vi "Factorial.vi"() -> ()   [LabVIEW 2022 SP3]
panel:
  out "N!":i64
  in  "N":i32
  # "Factorial:\nEnter a number N, to see the value of N!\nWhere N! = 1 * 2 * 3 * 4 * ... * N"
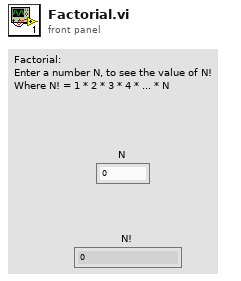
[diagram p1: front panel]
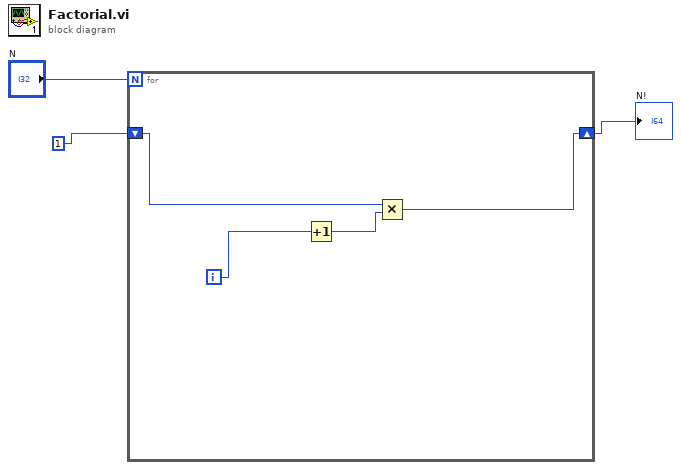
[diagram p0: block diagram]
diagram:
  n1 = for {
    N: "N" -> [_]
    shift-right: [w4] -> w1
    shift-left: 1 -> [w6]
    i -> [w7]
    n2 = Increment(x=w7) -> (x+1=w5:i64)
    n3 = Multiply(x=w6, y=w5) -> (x*y=w4:i64)
  }
  "N!" <- w1
